vi "Method.vi"(4 "Input B":refnum<class "Abs_Numeric.lvclass">, 5 "Input A":refnum<class "Abs_U64 Integer.lvclass">) -> (1 "Result":T1)   [LabVIEW 2021, in "Add_U64.lvclass"]
uses:
  Add_U64.lvclass
  Abs_Types/U64 Integer/Abs_U64 Integer.lvclass
  Abs_Types/Numeric/Abs_Numeric.lvclass
  Abs_Type.ctl
  C:/TSA/LV_Abstract/Source/Functions/Support/Function/Two Terminal/U64/AbsFunc_Two Term_U64.lvclass
  C:/Program Files (x86)/National Instruments/LabVIEW 2021/vi.lib/TSA/Abstract Data Classes/Abs_Types/U64 Integer/Abs_U64 Integer.lvclass
  Support/Function/Two Terminal/U64/AbsFunc_Two Term_U64.lvclass/AbsFunc_Two Term_U64.ctl
  Support/Function/Two Terminal/U64/Properties/Write Numeric A.vi
  Support/Function/Two Terminal/U64/Properties/Write Numeric B.vi
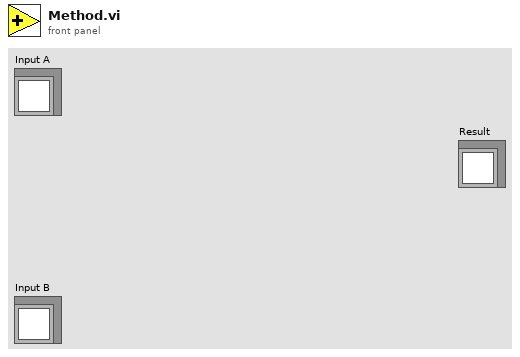
[diagram p1: front panel]
types:
  T1 = typedef "Add_U64.lvclass/Abs_Type.ctl" = refnum<class "Abs_U64 Integer.lvclass">
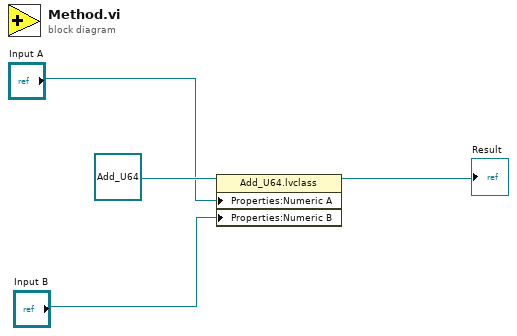
[diagram p0: block diagram]
diagram:
  n1 = property class="Add_U64.lvclass"(reference=refnum<class "Add_U64.lvclass"> refnum ("Functions.lvlib:Numeric.lvlib:Add_SGL.lvclass"), "Properties:Numeric A"="Input A", "Properties:Numeric B"="Input B") -> (reference out=→"Result":refnum<class "Add_U64.lvclass">)  [unwired: 1 in, 1 out]
